vi "PwrMtr_RSNRPZ_MatchIDNStr.vi"(8 "error in":errorcluster, 10 "IDNStr":string) -> (0 "error out":errorcluster, 2 "IDN match":bool, 3 "ClassLibraryFile":path)   [LabVIEW 2014]
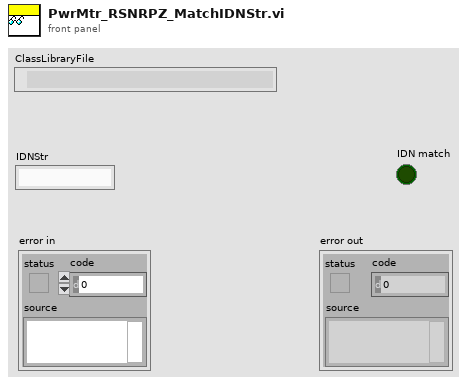
[diagram p1: front panel]
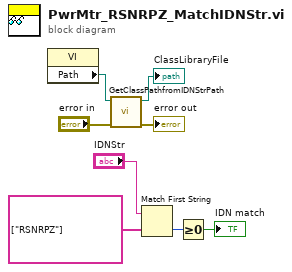
[diagram p0: block diagram]
diagram:
  n1 = property class="VI"() -> ("Path"=w6:path)  [unwired: 2 in, 2 out]
  n2 = call "GetClassPathfromIDNStrPath.vi"("error in (no error)"="error in", "Path in"=w6) -> ("error out"=→"error out":errorcluster, "Path out"=→"ClassLibraryFile":path)  [unwired: 8 in]
  n3 = Match First String(2:string[] ["RSNRPZ"] ("string array"), 3:"IDNStr") -> (0:w8:i32)  [unwired: 1 out]
  n4 = Greater Or Equal To 0?(x=w8) -> (x >= 0?=→"IDN match":bool)
